vi "ep_Flicker PT (1ch).vi"(0 "voltage waveform":waveform(dbl), 1 "init":bool, 5 "nominal frequency":enum16{"50 Hz", "60 Hz"}(ring), 7 "voltage system":enum16{"120 V", "230 V"}(ring), 9 "RMS (1/2) (half cycle)":cluster{"times":timestamp[], "RMS (1/2)":dbl[]}, 11 "nominal sampling rate [Hz]":dbl=1.0 format="%0.2f") -> (4 "instantaneous flicker Pinst (Output 5)":waveform(dbl))   [LabVIEW 2013, in "NI_EP_Power Quality.lvlib"]
doc: "This VI calculates flicker according to EN 61000-4-15, output 5 for one channel."
uses:
  <vilib>/addons/Electrical Power/PQ/NI_EP_Power Quality.lvlib
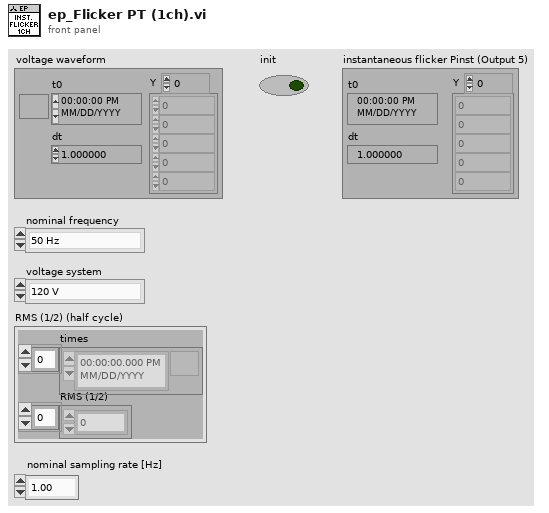
[diagram p1: front panel]
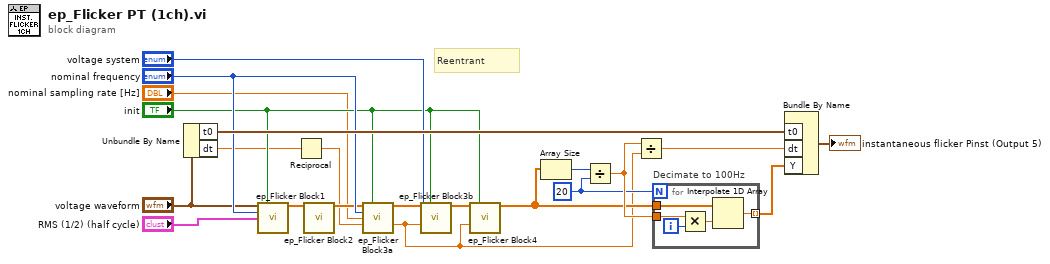
[diagram p0: block diagram]
diagram:
  w19 = 20 ("y")
  # "Reentrant"
  n1 = Unbundle By Name("voltage waveform") -> ("t0"=w21:timestamp, "dt"=w1:dbl)
  n2 = call <vilib>:"ep_Flicker Block1.vi"("voltage waveform"="voltage waveform", "init"="init", "nominal frequency"="nominal frequency", "RMS (1/2) (half cycle)"="RMS (1/2) (half cycle)") -> ("adapted voltage"=w7:dbl[])  [unwired: 11 in]
  n3 = Reciprocal(x=w1) -> (1/x=w4:dbl)
  n4 = call <vilib>:"ep_Flicker Block2.vi"("adapted voltage"=w7) -> ("squared voltage"=w8:dbl[])  [unwired: 14 in]
  n5 = call <vilib>:"ep_Flicker Block3a.vi"("squared voltage"=w8, "init"="init", "nominal frequency"="nominal frequency", "nominal sampling rate [Hz]"="nominal sampling rate [Hz]", "input sampling rate"=w4) -> ("filtered voltage"=w10:dbl[], "output sampling rate"=w3:dbl)  [unwired: 9 in]
  n6 = call <vilib>:"ep_Flicker Block3b.vi"("filtered voltage"=w10, "init"="init", "voltage system"="voltage system", "input sampling rate"=w3) -> ("weighted voltage fluctuation"=w9:dbl[])  [unwired: 11 in]
  n7 = call <vilib>:"ep_Flicker Block4.vi"("weighted voltage fluctuation"=w9, "init"="init", "input sampling rate"=w3) -> ("instant flicker"=w13:dbl[])  [unwired: 12 in]
  n8 = Array Size(array=w13) -> (size(s)=w18:i32)
  n9 = Divide(x=w18, y=w19) -> (x/y=w20:dbl)
  n10 = Divide(x=w20, y=w3) -> (x/y=w14:dbl)
  n11 = for "Decimate to 100Hz" {
    N: w19 -> [_]
    tunnel: w20 -> [w25]
    tunnel: w13 -> [w24]
    tunnel: [w22] -> w15 mode=indexing
    i -> [w26]
    n12 = Multiply(x=w25, y=w26) -> (x*y=w23:dbl)
    n13 = Interpolate 1D Array(1:w23, 2:w24) -> (0:w22:dbl)
  }
  n14 = Bundle By Name("t0"=w21, "dt"=w14, "Y"=w15) -> (→"instantaneous flicker Pinst (Output 5)":waveform(dbl))  [unwired: 1 in]
